vi "dataSocketPC.vi"(10 "目标经度":u16) -> ()   [LabVIEW 2012]
panel:
  in  "Target":string="dstp://localhost/longitude" caption="目标"
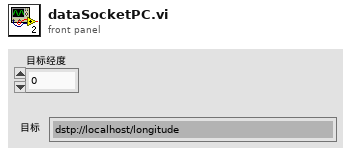
[diagram p1: front panel]
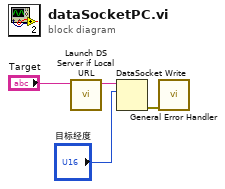
[diagram p0: block diagram]
diagram:
  n1 = call "Launch DS Server if Local URL.vi"("URL"="Target") -> ("Duplicate URL"=w2:string)  [unwired: 1 in, 5 out]
  n2 = DataSocket Write(10:"目标经度", 11:w2) -> (0:w1:errorcluster)  [unwired: 2 in, 2 out]
  n3 = call <vilib>:"General Error Handler.vi"("error in (no error)"=w1) -> ()  [unwired: 1 in, 14 out]
